vi "ReadSession.vi"(11 "IMAQdx in":refnum<class "IMAQdx.lvclass">) -> (2 "session":refnum<k21>, 3 "IMAQdx out":refnum<class "IMAQdx.lvclass">)   [LabVIEW 2010, in "IMAQdx.lvclass"]
uses:
  IMAQdx.lvclass
  IMAQdx.lvclass/IMAQdx.ctl
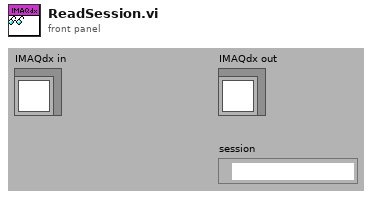
[diagram p1: front panel]
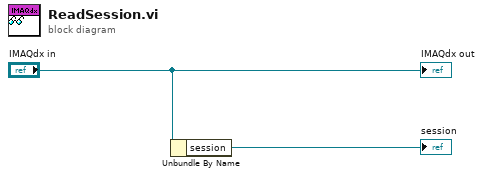
[diagram p0: block diagram]
diagram:
  n1 = Unbundle By Name("IMAQdx in") -> ("session"=→"session":refnum<k21>)
  "IMAQdx out" <- "IMAQdx in"
